vi "OCT Example.vi"() -> ()   [LabVIEW 2012]
uses:
  User Controls/Array Dimensions.ctl
  OCT States.ctl
  Non-User VIs/Error Checking/View Error Log Mode Functional Global.vi
  OpenCLV x64.lvlib
panel:
  in  "OpenCL Memory Type":enum16{"Global", "Local", "No optimization"}(ring)
  in  "Iterations":i32=5
  out "Average Time":dbl
  out "Phase":sgl[][](graph)
  out "Magnitude":sgl[][](graph)
  in  "Dimension In":T1={"Depth"=1, "Height"=1000, "Width"=1024} {"Width" min=1; "Height" min=1; "Depth" min=1}
  # "ms"
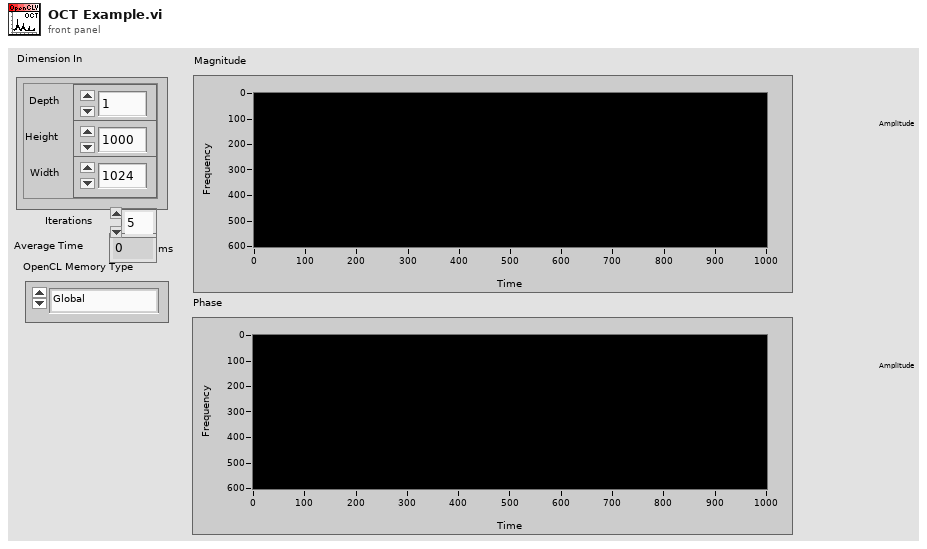
[diagram p1: front panel]
types:
  T1 = typedef "Array Dimensions.ctl" = cluster{"Depth":u64, "Height":u64, "Width":u64}
  T2 = typedef "OCT States.ctl" = enum16{"Allocate", "Pre-FFT No Optimization", "Pre-FFT Global Memory", "Pre-FFT Local Memory", "FFT", "Post FFT", "Read Data", "Clean-up"}
  T3 = typedef "OpenCLV x64.lvlib/Device ID.ctl" = u64
  T4 = typedef "OpenCLV x64.lvlib/Program Handle.ctl" = u64
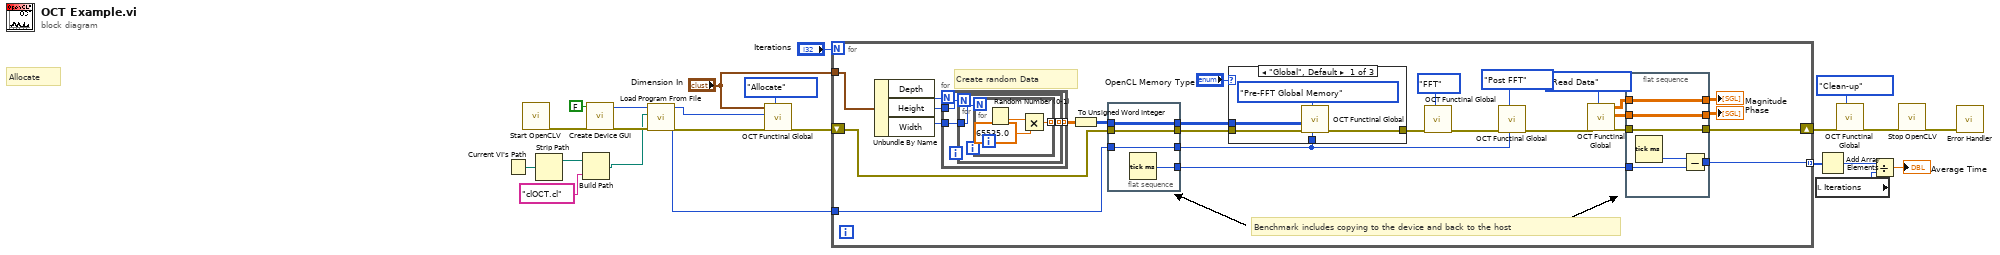
[diagram p0: block diagram]
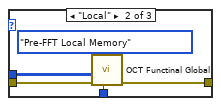
[diagram p2: hidden frame]
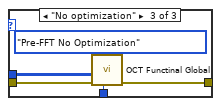
[diagram p3: hidden frame]
diagram:
  # "Allocate"
  n1 = Current VI's Path() -> (path=w18:path)
  n2 = call "Start OpenCLV.vi"() -> ("Error Out"=w23:errorcluster)  [unwired: 11 in]
  n3 = Strip Path(path=w18) -> (stripped path=w17:path)  [unwired: 1 out]
  n4 = Build Path(base path=w17, name or relative path="clOCT.cl") -> (appended path=w16:path)
  n5 = call "Create Device GUI.vi"("Error In"=w23, "Skip Configuration"=FALSE) -> ("error constant"=w21:errorcluster, "Device Reference"=w20:T3)  [unwired: 8 in]
  n6 = call "Load Program From File.vi"("Error In"=w21, "Program Path"=w16, "Device In"=w20) -> ("Error Out"=w14:errorcluster, "Program Handle"=w11:T4, "Device Out"=w13:T3)  [unwired: 6 in]
  n7 = call "OCT Functinal Global.vi"("FFT States"=OCT_States."Allocate", "Error In"=w14, "Device In"=w13, "Dimension In"="Dimension In") -> ("Error Out"=w5:errorcluster)  [unwired: 5 in, 2 out]
  n8 = for {
    N: "Iterations" -> [_]
    tunnel: w11 -> [w26]
    shift-right: [w30] -> w9
    shift-left: w5 -> [w27]
    tunnel: "Dimension In" -> [w38]
    tunnel: [w35] -> w2 mode=indexing
    # "Create random Data"
    # "Benchmark includes copying to the device and back to the host"
    n9 = Unbundle By Name(w38) -> ("Depth"=w42:u64, "Height"=w43:u64, "Width"=w41:u64)
    n10 = for {
      N: w42 -> [_]
      tunnel: w43 -> [w73]
      tunnel: w41 -> [w72]
      tunnel: [w71] -> w40 mode=indexing
      n11 = for {
        N: w73 -> [_]
        tunnel: w72 -> [w75]
        tunnel: [w74] -> w71 mode=indexing
        n12 = for {
          N: w75 -> [_]
          tunnel: [w77] -> w74 mode=indexing
          n13 = Random Number (0-1)() -> (number: 0 to 1=w78:dbl)
          n14 = Multiply(x=w78, y=65535.0) -> (x*y=w77:dbl)
        }
      }
    }
    n15 = To Unsigned Word Integer(number=w40) -> (unsigned 16bit integer=w39:u16[][][])
    n16 = flat-sequence {
      tunnel: w39 -> [w82]
      tunnel: [w82] -> w44
      tunnel: [w81] -> w36
      tunnel: [w80] -> w28
      tunnel: w27 -> [w80]
      tunnel: w26 -> [w79]
      tunnel: [w79] -> w25
      frame #0 {
        n17 = Tick Count (ms)() -> (millisecond timer value=w81:u32)
      }
    }
    n18 = case shown="\"Global\", Default" "OpenCL Memory Type" {
      tunnel: [w53 w58 w63] -> w49
      tunnel: w44 -> [w52 w56 w61]
      tunnel: w28 -> [w51 w57 w62]
      tunnel: w25 -> [w50 w59 w64]
      frame "Global", Default {
        n19 = call "OCT Functinal Global.vi"("Program Handle"=w50, "FFT States"=OCT_States."Pre-FFT Global Memory", "Error In"=w51, "Input U16 Data"=w52) -> ("Error Out"=w53:errorcluster)  [unwired: 5 in, 2 out]
      }
      frame "Local" {
        n20 = call "OCT Functinal Global.vi"("Program Handle"=w59, "FFT States"=OCT_States."Pre-FFT Local Memory", "Error In"=w57, "Input U16 Data"=w56) -> ("Error Out"=w58:errorcluster)  [unwired: 5 in, 2 out]
      }
      frame "No optimization" {
        n21 = call "OCT Functinal Global.vi"("Program Handle"=w64, "FFT States"=OCT_States."Pre-FFT No Optimization", "Error In"=w62, "Input U16 Data"=w61) -> ("Error Out"=w63:errorcluster)  [unwired: 5 in, 2 out]
      }
    }
    n22 = call "OCT Functinal Global.vi"("FFT States"=OCT_States."FFT", "Error In"=w49) -> ("Error Out"=w47:errorcluster)  [unwired: 7 in, 2 out]
    n23 = call "OCT Functinal Global.vi"("Program Handle"=w25, "FFT States"=OCT_States."Post FFT", "Error In"=w47) -> ("Error Out"=w37:errorcluster)  [unwired: 6 in, 2 out]
    n24 = call "OCT Functinal Global.vi"("FFT States"=OCT_States."Read Data", "Error In"=w37) -> ("Error Out"=w29:errorcluster, "Phase"=w33:sgl[][], "Magnitude"=w31:sgl[][])  [unwired: 7 in]
    n25 = flat-sequence {
      tunnel: w36 -> [w70]
      tunnel: [w69] -> w35
      tunnel: [w68] -> w34
      tunnel: w33 -> [w68]
      tunnel: [w67] -> w32
      tunnel: w31 -> [w67]
      tunnel: [w65] -> w30
      tunnel: w29 -> [w65]
      frame #0 {
        n26 = Tick Count (ms)() -> (millisecond timer value=w66:u32)
        n27 = Subtract(x=w66, y=w70) -> (x-y=w69:u32)
      }
    }
    "Phase" <- w34
    "Magnitude" <- w32
  }
  n28 = local read "Iterations"() -> (w12:i32)
  n29 = Add Array Elements(numeric array=w2) -> (sum=w1:u32)
  n30 = call "OCT Functinal Global.vi"("FFT States"=OCT_States."Clean-up", "Error In"=w9) -> ("Error Out"=w7:errorcluster)  [unwired: 7 in, 2 out]
  n31 = Divide(x=w1, y=w12) -> (x/y=→"Average Time":dbl)
  n32 = call "Stop OpenCLV.vi"("Error In"=w7) -> ("Error Out"=w6:errorcluster)  [unwired: 10 in]
  n33 = call-poly "Error Handler.vi"("Error In"=w6) -> ()  [unwired: 10 in, 1 out]
